vi "Suppress lines.vi"(8 "error in (no error)":errorcluster, 10 "Lines to suppress":u8[](array[numeric]), 11 "TTL in":refnum<class "TTL.lvclass">) -> (0 "error out":errorcluster, 3 "TTL out":refnum<class "TTL.lvclass">)   [LabVIEW 2011, in "TTL.lvclass"]
doc: "This VI sets a certain set of lines to zero, until the \"unsuppress\" VI is called again."
uses:
  TTL.lvclass
  TTL.lvclass/TTL.ctl
  <vilib>/DAQmx/write.llb/DAQmx Write (Digital 1D Bool NChan 1Samp 1Line).vi
  <vilib>/DAQmx/read.llb/DAQmx Read (Digital 1D Bool NChan 1Samp 1Line).vi
  <vilib>/DAQmx/miscellaneous.llb/DAQmx Fill In Error Info.vi
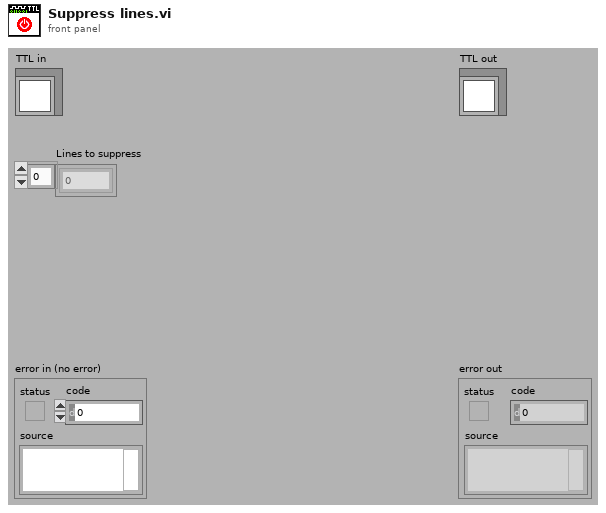
[diagram p1: front panel]
types:
  T1 = typedef "TTL.lvclass/TTL Status Data.ctl" = cluster{"Line states before suppression":bool[], "Suppressed lines":bool[]}
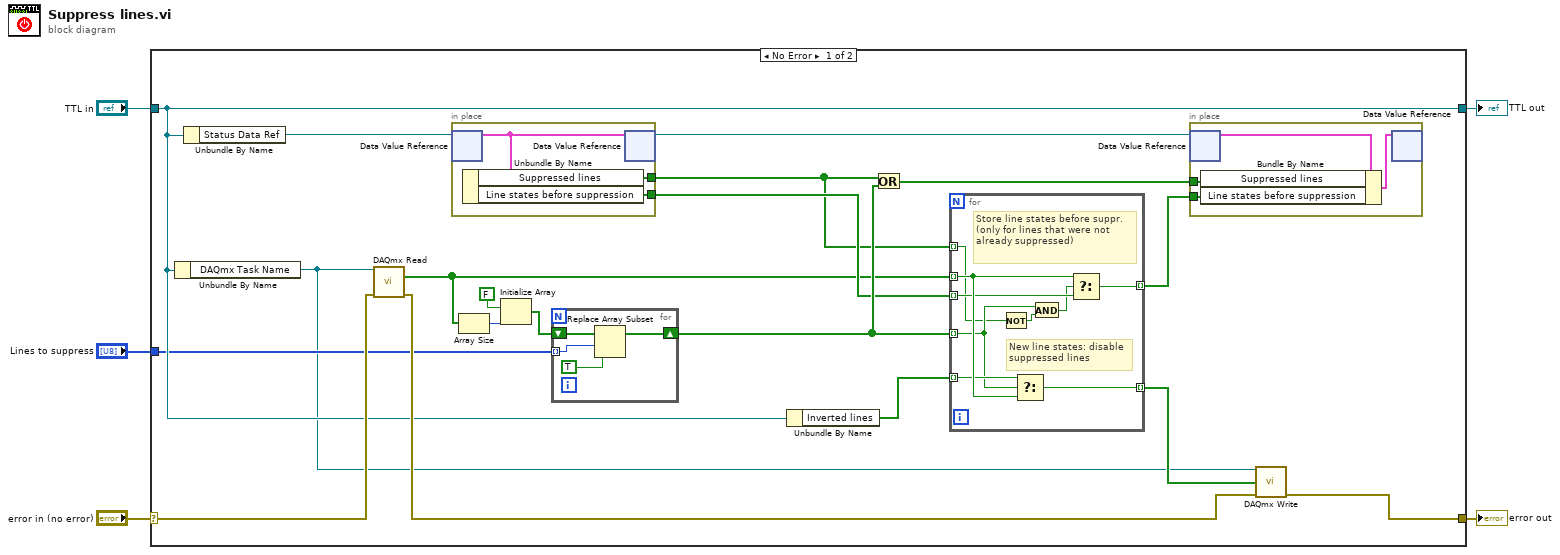
[diagram p0: block diagram]
diagram:
  n1 = case shown="No Error" "error in (no error)" {
    selector: "error in (no error)" -> [w23 w46]
    tunnel: [w21 w46] -> w4
    tunnel: [w12 w45] -> w2
    tunnel: "TTL in" -> [w12 w45]
    tunnel: "Lines to suppress" -> [w7 _]
    frame No Error {
      n2 = Unbundle By Name(w12) -> ("DAQmx Task Name"=w6:refnum<k21>)
      n3 = Unbundle By Name(w12) -> ("Status Data Ref"=w17:refnum<data-value>)
      n4 = call-poly <vilib>:"DAQmx Read.vi"("task/channels in"=w6, "error in"=w23) -> ("data"=w8:bool[], "error out"=w24:errorcluster)  [unwired: 11 in, 1 out]
      n5 = in-place {
        in-place-border: [w30] -> w9
        in-place-border: [w29] -> w10
        n6 = in-place-dvr #1(w17) -> (w31:T1)  [unwired: 1 out]
        n7 = Unbundle By Name(w31) -> ("Suppressed lines"=w30:bool[], "Line states before suppression"=w29:bool[])
        n8 = in-place-dvr #1(w31) -> (w14:refnum<data-value>)  [unwired: 1 out]
      }
      n9 = Array Size(array=w8) -> (size(s)=w20:i32)
      n10 = Initialize Array(FALSE, w20) -> (w18:bool[])
      n11 = for {
        tunnel: w7 -> [w34] mode=indexing
        shift-right: [w32] -> w13
        shift-left: w18 -> [w35]
        n12 = Replace Array Subset(array=w35, new element=TRUE, index=w34) -> (w32:bool[])
      }
      n13 = Unbundle By Name(w12) -> ("Inverted lines"=w11:bool[])
      n14 = Or(x=w9, y=w13) -> (x .or. y?=w16:bool[])
      n15 = for {
        tunnel: w13 -> [w38] mode=indexing
        tunnel: w8 -> [w43] mode=indexing
        tunnel: w10 -> [w40] mode=indexing
        tunnel: [w44] -> w15 mode=indexing
        tunnel: [w42] -> w22 mode=indexing
        tunnel: w11 -> [w41] mode=indexing
        tunnel: w9 -> [w36] mode=indexing
        # "Store line states before suppr. (only for lines that were not already suppressed)"
        # "New line states: disable\nsuppressed lines"
        n16 = Not(x=w36) -> (.not. x?=w37:bool)
        n17 = Select(t=w41, s=w38, f=w43) -> (s? t:f=w42:bool)
        n18 = And(x=w38, y=w37) -> (x .and. y?=w39:bool)
        n19 = Select(t=w43, s=w39, f=w40) -> (s? t:f=w44:bool)
      }
      n20 = in-place {
        in-place-border: w16 -> [w26]
        in-place-border: w15 -> [w25]
        n21 = in-place-dvr #2(w14) -> (w28:T1)  [unwired: 1 out]
        n22 = Bundle By Name(cluster=w28, "Suppressed lines"=w26, "Line states before suppression"=w25) -> (w27:T1)
        n23 = in-place-dvr #2(w27) -> ()  [unwired: 2 out]
      }
      n24 = call-poly <vilib>:"DAQmx Write.vi"("task/channels in"=w6, "data"=w22, "error in"=w24) -> ("error out"=w21:errorcluster)  [unwired: 10 in, 2 out]
    }
    frame Error {
    }
  }
  "error out" <- w4
  "TTL out" <- w2
